vi "getGoalAmount.vi"(7 "Category Name":string, 8 "error in (no error)":errorcluster, 9 "Month":T1, 10 "YYYY":i32, 11 "Account History in":refnum<class "Account History.lvclass">) -> (0 "error out":errorcluster, 2 "Amount":dbl, 3 "Account History out":refnum<class "Account History.lvclass">)   [LabVIEW 2018, in "Account History.lvclass"]
uses:
  Account History.lvclass
  Month.ctl
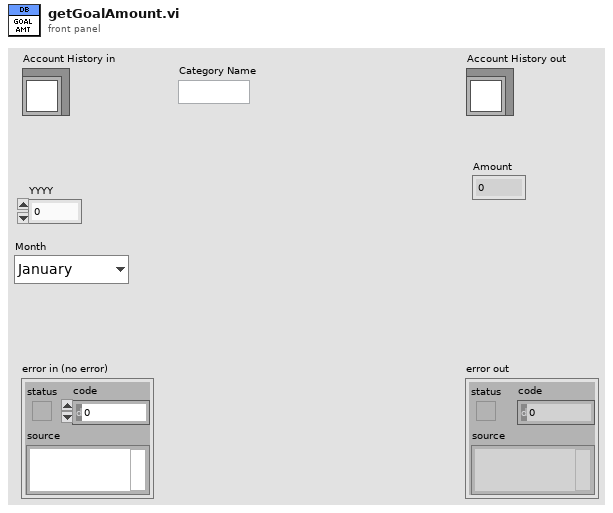
[diagram p1: front panel]
types:
  T1 = typedef "Account History.lvclass/Month.ctl" = enum16{"January", "February", "March", "April", "May", "June", "July", "August", "September", "October", "November", "December"}
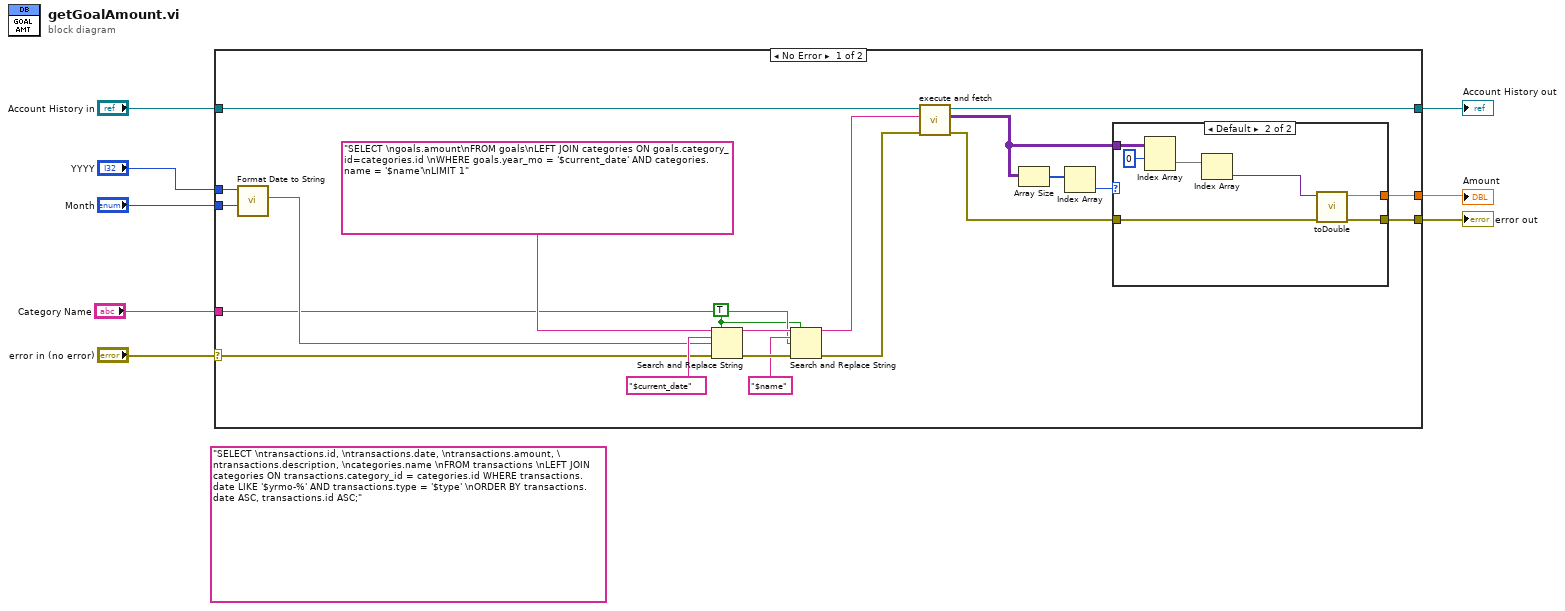
[diagram p0: block diagram]
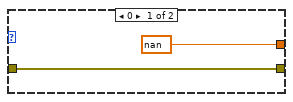
[diagram p2: hidden frame]
diagram:
  (unwired) "SELECT \ntransactions.id, \ntransactions.date, \ntransactions.amount, \ntransactions.description, \ncategories.name \nFROM transactions \nLEFT JOIN categories ON transactions.category_id = categories.id WHERE transactions.date LIKE '$yrmo-%' AND transactions.type = '$type' \nORDER BY transactions.date ASC, transactions.id ASC;"
  n1 = case shown="No Error" "error in (no error)" {
    selector: "error in (no error)" -> [w23 w40]
    tunnel: [w14 w40] -> w7
    tunnel: [w26 w39] -> w5
    tunnel: "Account History in" -> [w27 w39]
    tunnel: "YYYY" -> [w29 _]
    tunnel: "Month" -> [w28 _]
    tunnel: "Category Name" -> [w16 _]
    tunnel: [w9 _] -> w1
    frame No Error {
      w15 = TRUE ("replace all? (F)")
      n2 = call "Format Date to String.vi"("Month"=w28, "YYYY"=w29) -> ("Year-Mo"=w22:string)  [unwired: 9 in]
      n3 = Search and Replace String(replace all?=w15, input string="SELECT \ngoals.amount\nFROM goals\nLEFT JOIN categories ON goals.category_id=categories.id \nWHERE goals.year_mo = '$current_date' AND categories.name = '$name'\nLIMIT 1", search string="$current_date", replace string=w22, error in=w23) -> (result string=w20:string, error out=w21:errorcluster)  [unwired: 3 in, 2 out]
      n4 = Search and Replace String(replace all?=w15, input string=w20, search string="$name", replace string=w16, error in=w21) -> (result string=w19:string, error out=w18:errorcluster)  [unwired: 3 in, 2 out]
      n5 = call "execute and fetch.vi"("error in (no error)"=w18, "SQL query"=w19, "Database in"=w27) -> ("error out"=w13:errorcluster, "recordset data"=w12:variant[][], "Database out"=w26:refnum<class "Account History.lvclass">)  [unwired: 5 in, 1 out]
      n6 = Array Size(array=w12) -> (size(s)=w11:i32[])
      n7 = Index Array(array=w11) -> (element=w10:i32)  [unwired: 1 in]
      n8 = case shown="Default" w10 {
        tunnel: [w31 w33] -> w14
        tunnel: w13 -> [w31 w34]
        tunnel: w12 -> [_ w36]
        tunnel: [nan ("type") w32] -> w9
        frame 0 {
        }
        frame Default {
          n9 = Index Array(array=w36, index (row)=0) -> (element=w38:variant[])  [unwired: 1 in]
          n10 = Index Array(array=w38) -> (element=w35:variant)  [unwired: 1 in]
          n11 = call "toDouble.vi"("error in (no error)"=w34, "Value"=w35) -> ("error out"=w33:errorcluster, "type"=w32:dbl)  [unwired: 8 in]
        }
      }
    }
    frame Error {
    }
  }
  "error out" <- w7
  "Account History out" <- w5
  "Amount" <- w1
